vi "MaxTime.vi"(9 "maxTime":u32, 11 "Reset?":bool) -> (4 "Finished?":bool)   [LabVIEW 2014]
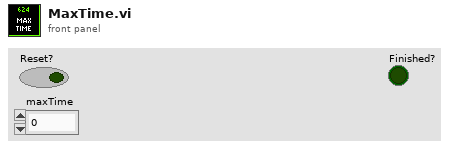
[diagram p1: front panel]
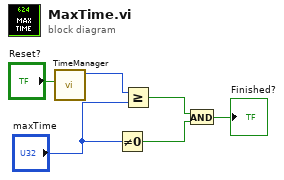
[diagram p0: block diagram]
diagram:
  n1 = call "TimeManager.vi"("Reset?"="Reset?") -> ("Time Since Reset"=w5:u32)  [unwired: 9 in, 1 out]
  n2 = Not Equal To 0?(x="maxTime") -> (x != 0?=w2:bool)
  n3 = Greater Or Equal?(x=w5, y="maxTime") -> (x >= y?=w3:bool)
  n4 = And(x=w3, y=w2) -> (x .and. y?=→"Finished?":bool)
